vi "checksum.vi"(1 "data":u8[](array[numeric])) -> (0 "checksum":u8)   [LabVIEW 2018]
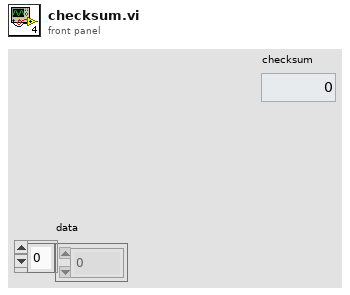
[diagram p1: front panel]
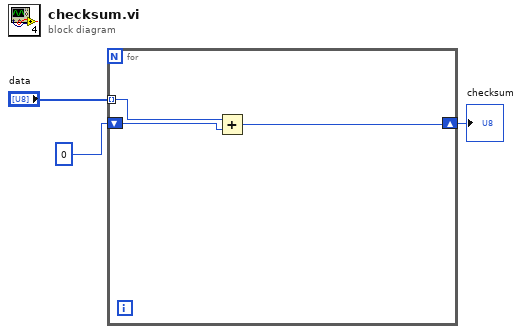
[diagram p0: block diagram]
diagram:
  n1 = for {
    shift-right: [w4] -> w1
    shift-left: u8 0 -> [w5]
    tunnel: "data" -> [w6] mode=indexing
    n2 = Add(x=w6, y=w5) -> (x+y=w4:u8)
  }
  "checksum" <- w1
